vi "Turn Off.vi"(8 "error in (no error)":errorcluster, 11 "Lamp in":refnum<class "Lamp.lvclass">) -> (0 "error out":errorcluster, 3 "Lamp out":refnum<class "Lamp.lvclass">)   [LabVIEW 2018, in "Lamp.lvclass"]
uses:
  Lamp.lvclass
  Lamp.lvclass/Lamp.ctl
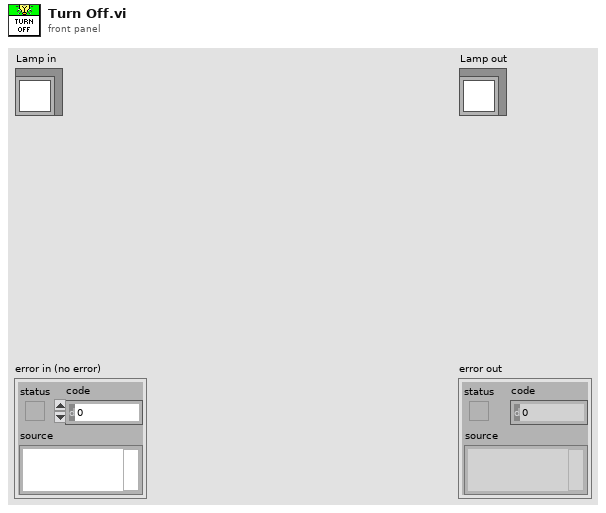
[diagram p1: front panel]
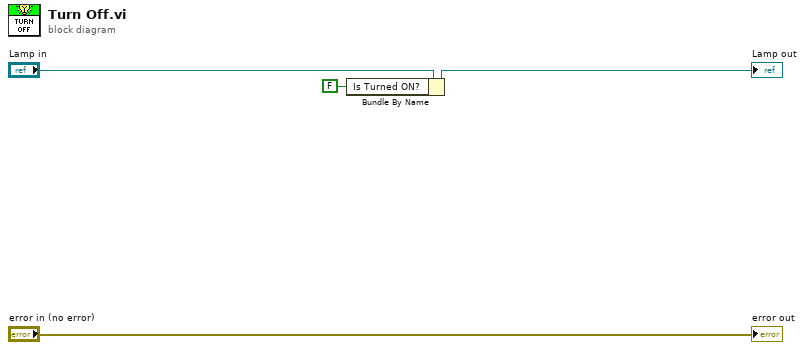
[diagram p0: block diagram]
diagram:
  n1 = Bundle By Name(cluster="Lamp in", "Is Turned ON?"=FALSE) -> (→"Lamp out":refnum<class "Lamp.lvclass">)
  "error out" <- "error in (no error)"
